vi "To String.vi"(8 "error in (no error)":errorcluster, 11 "String in":refnum<class "String.lvclass">) -> (0 "error out":errorcluster, 2 "String":string)   [LabVIEW 2020, in "Data.lvlib" / "String.lvclass"]
doc: "Convert 'Generic Data in' to a string.\nThe default implementation convert the data to an XML string."
uses:
  String.lvclass
  String.lvclass/String.ctl
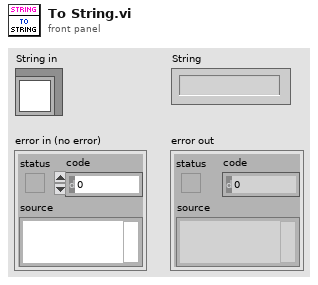
[diagram p1: front panel]
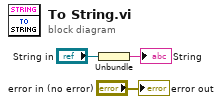
[diagram p0: block diagram]
diagram:
  n1 = Unbundle("String in") -> (→"String":string)
  "error out" <- "error in (no error)"
